vi "Get Version.vi"(6 "timeout (ms)":i32=5000, 8 "error in":errorcluster, 11 "gRPC ID":T2) -> (0 "error out":errorcluster, 2 "Version":T1, 3 "gRPC ID out":T2)   [LabVIEW 2021, in "CIFCorePluginWrapper.lvlib"]
uses:
  CIFCorePluginWrapper.lvlib
  <vilib>/gRPC/LabVIEW gRPC Library/Shared/grpcId.ctl
  CIFCoreCommon/Typedef/Version.ctl
  CIFCorePlugin_client/CIFCorePlugin_client.lvlib
  <vilib>/gRPC/LabVIEW gRPC Library/grpc-lvsupport-release.lvlib
  CIFCoreCommon/CIFCoreCommon.lvlib
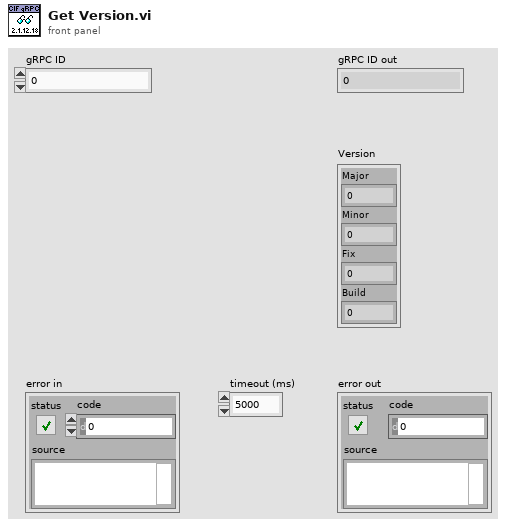
[diagram p1: front panel]
types:
  T1 = typedef "CIFCoreCommon.lvlib/Version.ctl" = cluster{"Major":i32, "Minor":i32, "Fix":i32, "Build":i32}
  T2 = typedef "grpc-lvsupport-release.lvlib/grpcId.ctl" = u64
  T3 = typedef "CIFCorePlugin_client.lvlib/cif_plugincore_Version.ctl" = cluster{"major":u32, "minor":u32, "fix":u32, "build":u32}
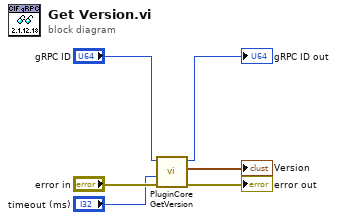
[diagram p0: block diagram]
diagram:
  n1 = call "PluginCore GetVersion.vi"("error in"="error in", "timeout (ms)"="timeout (ms)", "gRPC ID"="gRPC ID") -> ("error out"=→"error out":errorcluster, "Response Data"=→"Version":T3, "gRPC ID out"=→"gRPC ID out":T2)  [unwired: 6 in]
